vi "Get Project Hierarchy.vi"(8 "error in (no error)":errorcluster, 11 "Project Path":path) -> (0 "error out":errorcluster, 1 "Actual Locations":path[](array[path]), 3 "Expected Locations":path[](array[path]))   [LabVIEW 2023]
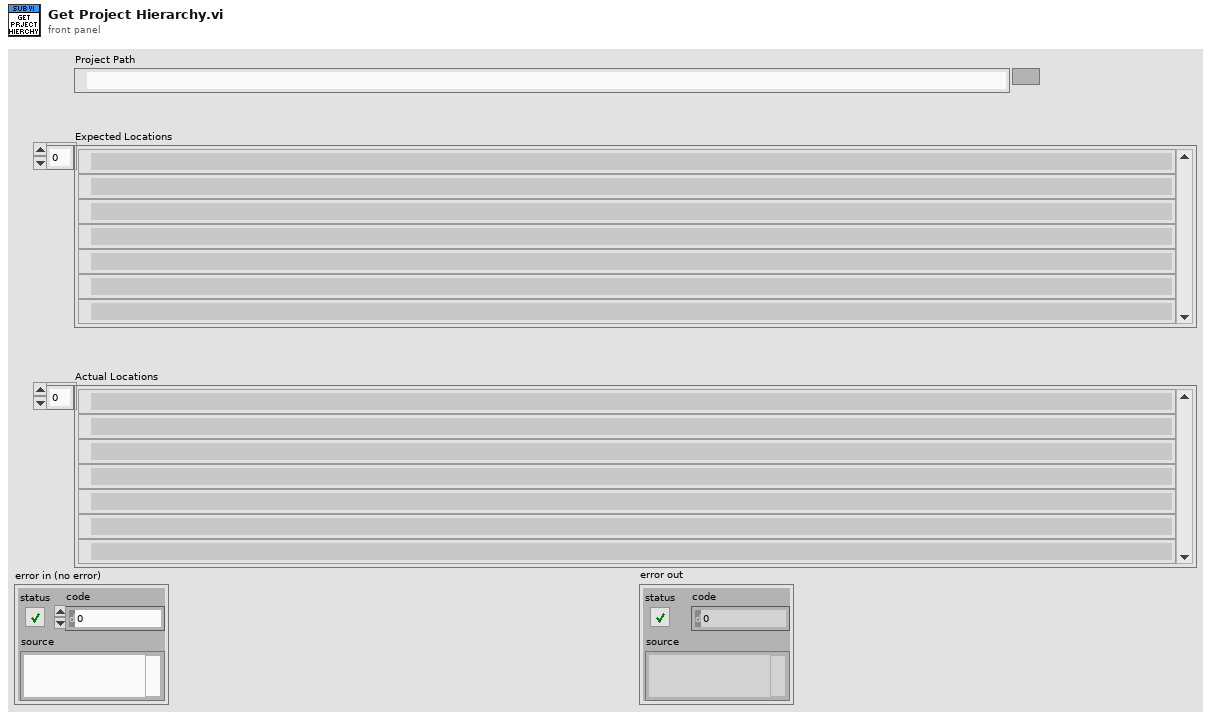
[diagram p1: front panel]
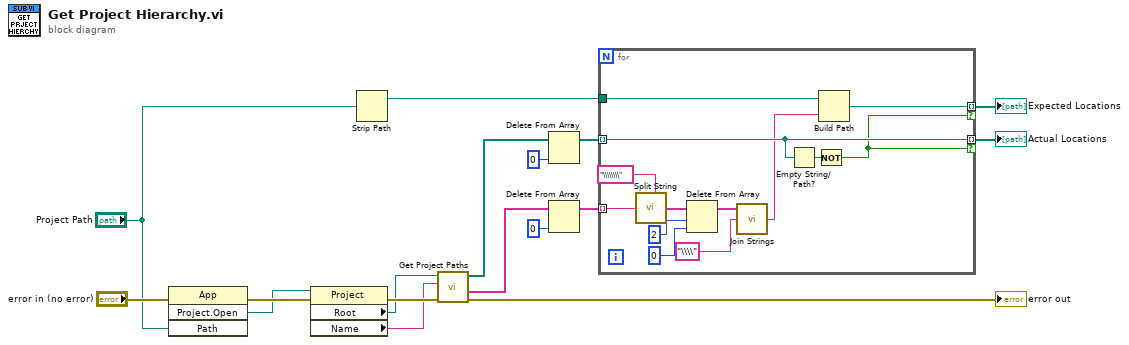
[diagram p0: block diagram]
diagram:
  n1 = invoke class="App" method="Project.Open"(error in="error in (no error)", "Path"="Project Path") -> (error out=w15:errorcluster, "Project:Open"=w13:refnum<vi>)  [unwired: 2 in, 2 out]
  n2 = property class="Project"(reference=w13, error in=w15) -> (error out=w17:errorcluster, "Root"=w12:refnum<vi>, "Name"=w11:string)  [unwired: 1 out]
  n3 = Strip Path(path="Project Path") -> (stripped path=w9:path)  [unwired: 1 out]
  n4 = call "Get Project Paths.vi"("error in (no error)"=w17, "Name"=w11, "ProjectItem refnum"=w12) -> ("error out"=→"error out":errorcluster, "Virtual Path"=w6:string[], "Path on Disk"=w3:path[])  [unwired: 6 in]
  n5 = Delete From Array(array=w3, index=0) -> (array with subset deleted=w2:path[])  [unwired: 1 in, 1 out]
  n6 = Delete From Array(array=w6, index=0) -> (array with subset deleted=w1:string[])  [unwired: 1 in, 1 out]
  n7 = for {
    tunnel: w2 -> [w22] mode=indexing
    tunnel: w1 -> [w19] mode=indexing
    tunnel: [w22] -> w7 mode=indexing if=w18
    tunnel: w9 -> [w25]
    tunnel: [w21] -> w8 mode=indexing if=w18
    n8 = call <vilib>:"Split String.vi"("Split Pattern"="\\\\\\\\", "Input String"=w19) -> ("Split String"=w29:string[])  [unwired: 5 in]
    n9 = Delete From Array(array=w29, length=2 ("index"), index=0) -> (array with subset deleted=w28:string[])  [unwired: 1 out]
    n10 = call <vilib>:"Join Strings.vi"("Separator (,)"="\\\\" ("Split Pattern"), "Strings In"=w28) -> ("String"=w20:string)  [unwired: 1 in]
    n11 = Empty String/Path?(string/path=w22) -> (empty?=w30:bool)
    n12 = Not(x=w30) -> (.not. x?=w18:bool)
    n13 = Build Path(base path=w25, name or relative path=w20) -> (appended path=w21:path)
  }
  "Expected Locations" <- w8
  "Actual Locations" <- w7
